vi "Pretty Print Level.vi"(8 "error in (no error)":errorcluster, 10 "Action":enum16{"Increment", "Decrement", "Get", "Reset"}(ring)) -> (0 "error out":errorcluster, 2 "Numeric":i32)   [LabVIEW 2017, in "LVJSON.lvlib"]
uses:
  LVJSON.lvlib
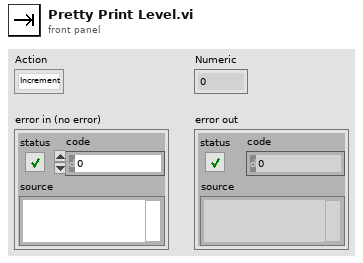
[diagram p1: front panel]
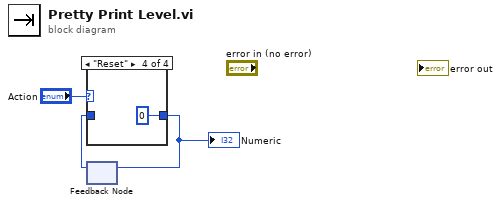
[diagram p0: block diagram]
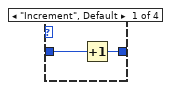
[diagram p2: hidden frame]
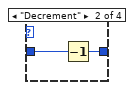
[diagram p3: hidden frame]
diagram:
  n1 = feedback #1() -> (w1:i32)  [unwired: 1 in]
  n2 = case shown="\"Reset\"" "Action" {
    tunnel: [w4 w6 w8 0] -> w2
    tunnel: w1 -> [w5 w7 w8 _]
    frame "Increment", Default {
      n3 = Increment(x=w5) -> (x+1=w4:i32)
    }
    frame "Decrement" {
      n4 = Decrement(x=w7) -> (x-1=w6:i32)
    }
    frame "Get" {
    }
    frame "Reset" {
    }
  }
  "Numeric" <- w2
  n5 = feedback-in #1(w2) -> ()
